vi "getClassHierarchyVersions.vi"(8 "error in":errorcluster, 10 "className":string) -> (0 "error out":errorcluster, 2 "allClassVersionNumbers":T1(array[cluster]))   [LabVIEW 2020, in "JKI JSON Object Serialization.lvlib" / "OOP_Utility.lvlib" / "Reflection.lvclass"]
doc: "Get the class hierarchy version numbers for the specified class. The first element of the output array is the version number for the input class; the last element is for the top most parent class. Input className can include or exclude the '.lvclass' extension. \n\nGCraftsman JSON Object Serialization Toolkit\nwww.GCraftsman.com\nCopyright (c) 2017, GCraftsman"
uses:
  Reflection.lvclass
  reflectionPoolAction.ctl
  Reflection.lvclass/Reflection.ctl
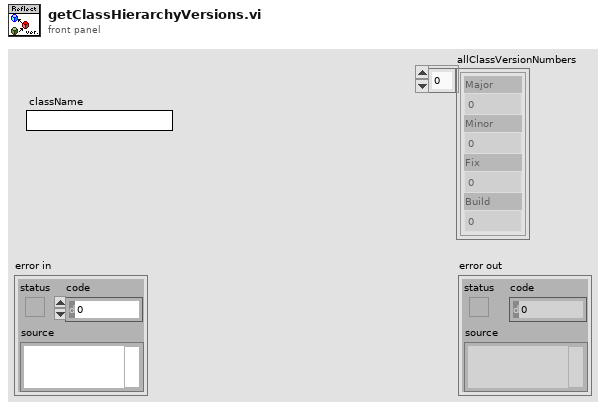
[diagram p1: front panel]
types:
  T1 = cluster{"Major":u16, "Minor":u16, "Fix":u16, "Build":u16}[]
  T2 = typedef "JKI JSON Object Serialization.lvlib/OOP_Utility.lvlib/Reflection.lvclass/reflectionPoolAction.ctl" = enum16{"<select>", "getPrivateData", "getClassHierarchy", "getClassVersions", "getAllClasses"}
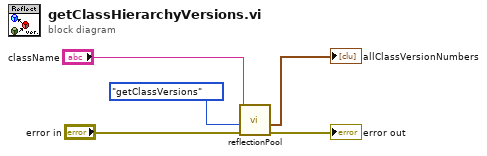
[diagram p0: block diagram]
diagram:
  n1 = call "reflectionPool.vi"("error in (no error)"="error in", "action"=reflectionPoolAction."getClassVersions", "class name"="className") -> ("error out"=→"error out":errorcluster, "class version numbers"=→"allClassVersionNumbers":T1)  [unwired: 3 in, 4 out]
